vi "generateTimeVector.vi"(2 "sampling time":dbl, 3 "record length":i16) -> (0 "time vector":dbl[](array[numeric]))   [LabVIEW 2010]
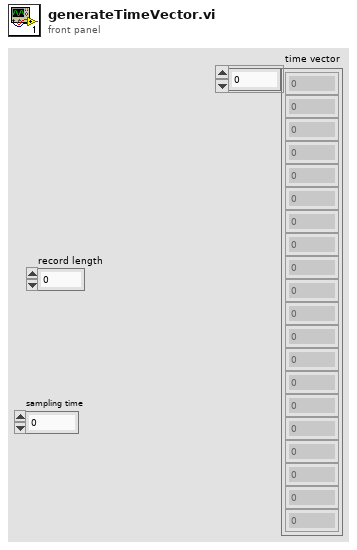
[diagram p1: front panel]
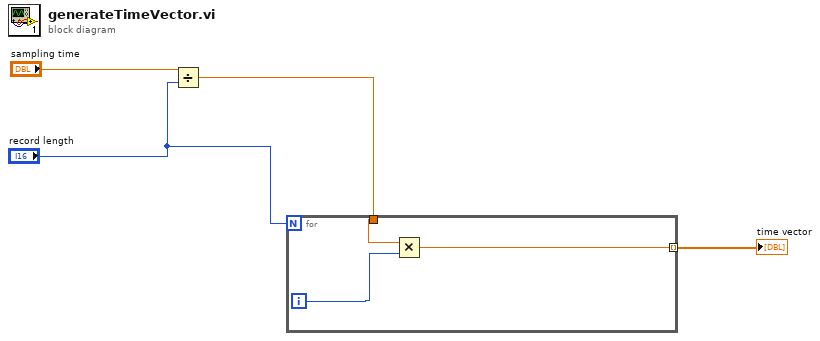
[diagram p0: block diagram]
diagram:
  n1 = Divide(x="sampling time", y="record length") -> (x/y=w3:dbl)
  n2 = for {
    N: "record length" -> [_]
    tunnel: w3 -> [w7]
    tunnel: [w6] -> w2 mode=indexing
    i -> [w5]
    n3 = Multiply(x=w7, y=w5) -> (x*y=w6:dbl)
  }
  "time vector" <- w2
